vi "Tx Event Clear.vi"(8 "error in (no error)":errorcluster, 11 "Tx Event":T1) -> (0 "error out":errorcluster)   [LabVIEW 2020, in "985x Support Addon Engine.lvlib"]
uses:
  985x Support Addon Engine.lvlib
  Types/Tx Event Session.ctl
  Types/FPGA Refnum.ctl
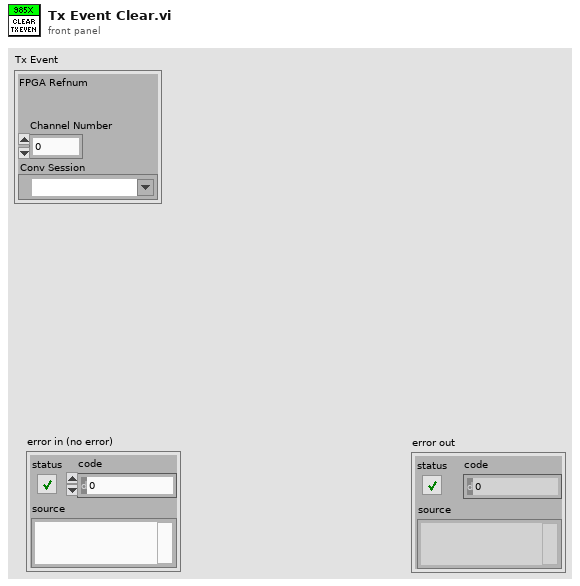
[diagram p1: front panel]
types:
  T1 = typedef "985x Support Addon Engine.lvlib/Tx Event Session.ctl" = cluster{"FPGA Refnum":T2, "Channel Number":u32, "Conv Session":refnum<k21>}
  T2 = typedef "985x Support Addon Engine.lvlib/FPGA Refnum.ctl" = refnum<k20>
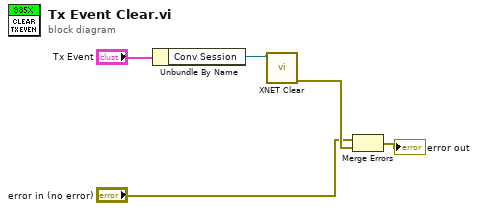
[diagram p0: block diagram]
diagram:
  n1 = Unbundle By Name("Tx Event") -> ("Conv Session"=w1:refnum<k21>)
  n2 = call <vilib>:"XNET Clear.vi"("session in"=w1) -> ("error out"=w5:errorcluster)  [unwired: 14 in]
  n3 = Merge Errors("error in (no error)", w5) -> (→"error out":errorcluster)
